vi "Curtin1_AddSettings.vi"(8 "Date?":bool, 9 "Check?":enum16{"Ignore", "Check", "Replace"}(ring)=enum."Check", 10 "Template":string, 11 "Settings in":T2={"Name of test"="", "Date"=timestamp(0 s since 1904-01-01), "Location"="", "Template"="", "Soundcard"="", "resolution"=0, "Sampling rate"=0, "Ch1 Gain "=25.0, "Ch2 Gain"=10.0, "Sample time (s)"=0.0, "Pre-trigger (s)"=0.0, "Hammer Threshold"=0.0, "Positions"=0, "Taps/Position"=0, "Set Names"="", "Freq resolution"=0.0, "Hammer cutoff"=0.0, "Mic cutoff"=0.0, "Double bounce "=0.0, "Hammer Cal"=0.0, "dB Offset"=0.0, "Accel Cal"=0.0, "Vibrometer Cal"=0.0, "Mic Cal"=0.0, "Output"=0, "Voltage Cal"=1.0, "Vibrometer Port"="ASRL27::INSTR", "Range"=4, "High Pass"=2, "Bandwidth"=4, "X Range"=[], "Y Range"=[], "dB Spread"=0.0, "Trigger"=0, "Ch_1"=25, "Ch_2"=25, "flip?"=FALSE, "60Hz"=FALSE, "Time offset"=0.0, "Piezo Cal"=1.0, "Default Notes"="", "Tom"=FALSE} {"Ch_2" min=1 step=1; "Ch_1" min=1 max=100 step=1; "Trigger" items=["Hammer (force)", "Self-tap", "Spacebar"]; "Bandwidth" items=["1 kHz"=1, "5 kHz"=5, "10 kHz"=10, "25 kHz"=25, "50 kHz"=50, "100 kHz"=100]; "High Pass" items=["Off", "13 Hz", "104 Hz"]; "Range" items=["10 mm/s"=1, "20 mm/s"=2, "50 mm/s"=5, "100 mm/s"=10, "200 mm/s"=20, "500 mm/s"=50, "1 m/s"=100, "2 m/s"=200]; "Output" items=["Accelerometer", "Speed (from acceleration)", "Microphone", "Vibrometer", "Piezo"]; "Voltage Cal" format="%#_13g"; "Ch2 Gain" format="%#_13g"; "Ch1 Gain" format="%#_13g"; "Double bounce" min=0.0; "Mic cutoff" min=0.0 format="%#_4g"; "Hammer cutoff" min=0.0 format="%#_4g"; "Freq resolution" min=0.0; "Pre-trigger (s)" format="%#_13g"; "Date" format="%<%H:%M\n%d/%m/%y>T"; "resolution" items=["16 bit"=16, "24 bit"=24, "32 bit"=32]; "Sampling rate" items=["22050 samp/s"=22050, "44100 samp/s"=44100, "48000 samp/s"=48000]}) -> (0 "text":string, 3 "Settings Out":T2={"Name of test"="", "Date"=timestamp(0 s since 1904-01-01), "Location"="", "Template"="", "Soundcard"="", "resolution"=0, "Sampling rate"=0, "Ch1 Gain "=25.0, "Ch2 Gain"=10.0, "Sample time (s)"=0.0, "Pre-trigger (s)"=0.0, "Hammer Threshold"=0.0, "Positions"=0, "Taps/Position"=0, "Set Names"="", "Freq resolution"=0.0, "Hammer cutoff"=0.0, "Mic cutoff"=0.0, "Double bounce "=0.0, "Hammer Cal"=0.0, "dB Offset"=0.0, "Accel Cal"=0.0, "Vibrometer Cal"=0.0, "Mic Cal"=0.0, "Output"=0, "Voltage Cal"=1.0, "Vibrometer Port"="ASRL27::INSTR", "Range"=4, "High Pass"=2, "Bandwidth"=4, "X Range"=[], "Y Range"=[], "dB Spread"=0.0, "Trigger"=0, "Ch_1"=25, "Ch_2"=25, "flip?"=FALSE, "60Hz"=FALSE, "Time offset"=0.0, "Piezo Cal"=1.0, "Default Notes"="", "Tom"=FALSE} {"Ch_2" min=1 step=1; "Ch_1" min=1 max=100 step=1; "Trigger" items=["Hammer (force)", "Self-tap", "Spacebar"]; "Bandwidth" items=["1 kHz"=1, "5 kHz"=5, "10 kHz"=10, "25 kHz"=25, "50 kHz"=50, "100 kHz"=100]; "High Pass" items=["Off", "13 Hz", "104 Hz"]; "Range" items=["10 mm/s"=1, "20 mm/s"=2, "50 mm/s"=5, "100 mm/s"=10, "200 mm/s"=20, "500 mm/s"=50, "1 m/s"=100, "2 m/s"=200]; "Output" items=["Accelerometer", "Speed (from acceleration)", "Microphone", "Vibrometer", "Piezo"]; "Voltage Cal" format="%#_13g"; "Ch2 Gain" format="%#_13g"; "Ch1 Gain" format="%#_13g"; "Double bounce" min=0.0; "Mic cutoff" min=0.0 format="%#_4g"; "Hammer cutoff" min=0.0 format="%#_4g"; "Freq resolution" min=0.0; "Pre-trigger (s)" format="%#_13g"; "Date" format="%<%H:%M\n%d/%m/%y>T"; "resolution" items=["16 bit"=16, "24 bit"=24, "32 bit"=32]; "Sampling rate" items=["22050 samp/s"=22050, "44100 samp/s"=44100, "48000 samp/s"=48000]})   [LabVIEW 2022 SP3]
uses:
  PreferencesControl.ctl
panel:
  out "x = y?":T1
  # "Hz"
  # "dB"
  # "dB"
  # "sec"
  # "sec"
  # "mV/Pa"
  # "mV/m/s2"
  # "mV/mm/s"
  # "V/N"
  # "sec"
  # "sec"
  # "mV/N"
  # "a.u."
  # "a.u."
  # "sec"
  # "Hz"
  # "dB"
  # "dB"
  # "sec"
  # "sec"
  # "mV/Pa"
  # "mV/m/s2"
  # "mV/mm/s"
  # "V/N"
  # "sec"
  # "sec"
  # "mV/N"
  # "a.u."
  # "a.u."
  # "sec"
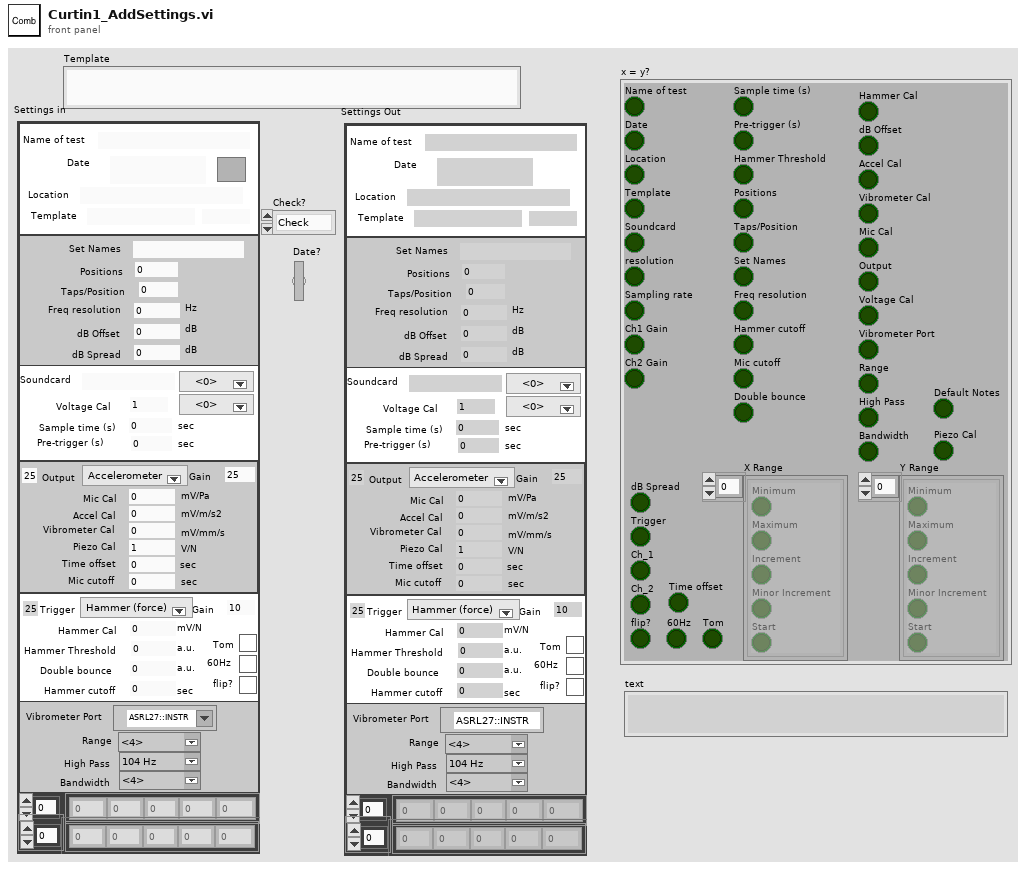
[diagram p1: front panel]
types:
  T1 = cluster{"Name of test":bool, "Date":bool, "Location":bool, "Template":bool, "Soundcard":bool, "resolution":bool, "Sampling rate":bool, "Ch1 Gain ":bool, "Ch2 Gain":bool, "Sample time (s)":bool, "Pre-trigger (s)":bool, "Hammer Threshold":bool, "Positions":bool, "Taps/Position":bool, "Set Names":bool, "Freq resolution":bool, "Hammer cutoff":bool, "Mic cutoff":bool, "Double bounce ":bool, "Hammer Cal":bool, "dB Offset":bool, "Accel Cal":bool, "Vibrometer Cal":bool, "Mic Cal":bool, "Output":bool, "Voltage Cal":bool, "Vibrometer Port":bool, "Range":bool, "High Pass":bool, "Bandwidth":bool, "X Range":cluster{"Minimum":bool, "Maximum":bool, "Increment":bool, "Minor Increment":bool, "Start":bool}[], "Y Range":cluster{"Minimum":bool, "Maximum":bool, "Increment":bool, "Minor Increment":bool, "Start":bool}[], "dB Spread":bool, "Trigger":bool, "Ch_1":bool, "Ch_2":bool, "flip?":bool, "60Hz":bool, "Time offset":bool, "Piezo Cal":bool, "Default Notes":bool, "Tom":bool}
  T2 = typedef "PreferencesControl.ctl" = cluster{"Name of test":string, "Date":timestamp, "Location":string, "Template":string, "Soundcard":string, "resolution":u16, "Sampling rate":u16, "Ch1 Gain ":dbl, "Ch2 Gain":dbl, "Sample time (s)":dbl, "Pre-trigger (s)":dbl, "Hammer Threshold":dbl, "Positions":i16, "Taps/Position":i16, "Set Names":string, "Freq resolution":dbl, "Hammer cutoff":dbl, "Mic cutoff":dbl, "Double bounce ":dbl, "Hammer Cal":dbl, "dB Offset":dbl, "Accel Cal":dbl, "Vibrometer Cal":dbl, "Mic Cal":dbl, "Output":u16, "Voltage Cal":dbl, "Vibrometer Port":refnum<visa-resource-name>, "Range":u16, "High Pass":u16, "Bandwidth":u16, "X Range":cluster{"Minimum":dbl, "Maximum":dbl, "Increment":dbl, "Minor Increment":dbl, "Start":dbl}[], "Y Range":cluster{"Minimum":dbl, "Maximum":dbl, "Increment":dbl, "Minor Increment":dbl, "Start":dbl}[], "dB Spread":dbl, "Trigger":u16, "Ch_1":u8, "Ch_2":u8, "flip?":bool, "60Hz":bool, "Time offset":dbl, "Piezo Cal":dbl, "Default Notes":string, "Tom":bool}
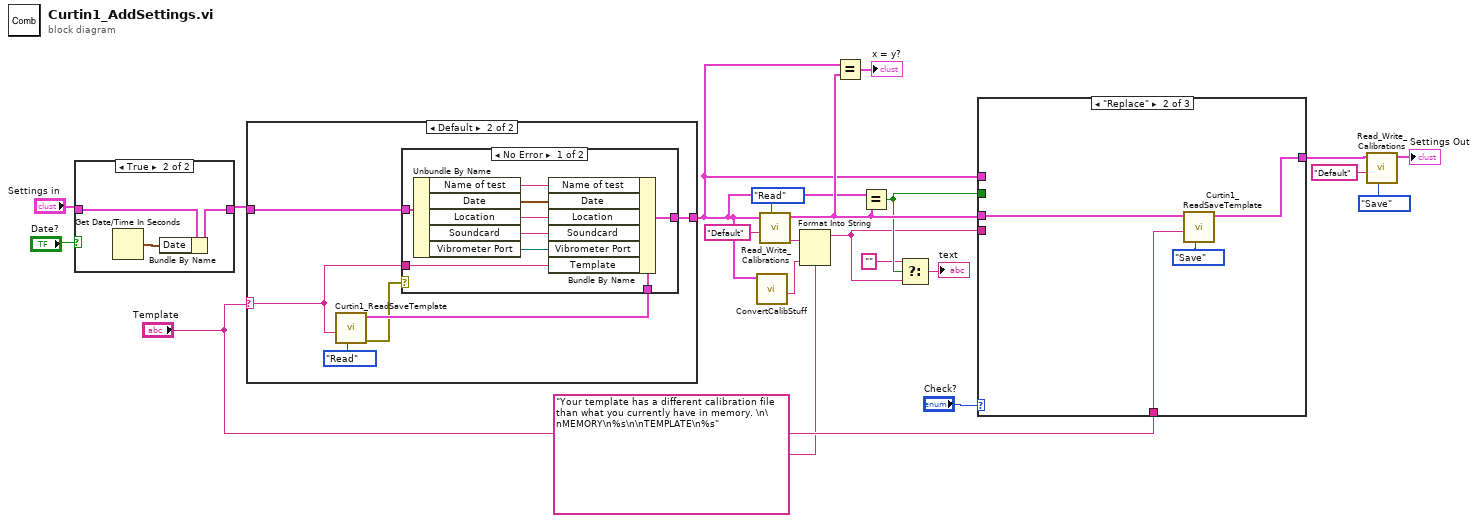
[diagram p0: block diagram]
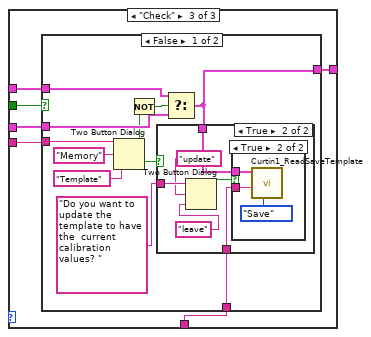
[diagram p3: hidden frame]
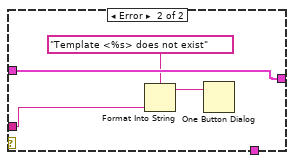
[diagram p9: hidden frame]
diagram:
  n1 = case shown="True" "Date?" {
    tunnel: "Settings in" -> [w22 w24]
    tunnel: [w22 w23] -> w18
    frame False {
    }
    frame True {
      n2 = Get Date/Time In Seconds() -> (seconds since 1Jan1904=w25:timestamp)
      n3 = Bundle By Name(cluster=w24, "Date"=w25) -> (w23:T2)
    }
  }
  n4 = case shown="Default" "Template" {
    selector: "Template" -> [_ w28]
    tunnel: [w26 w32] -> w8
    tunnel: w18 -> [w26 w31]
    frame "" {
    }
    frame Default {
      n5 = call "Curtin1_ReadSaveTemplate.vi"("Task"=enum16{"Save", "Read", "List"}."Read", "Template"=w28) -> ("error out"=w27:errorcluster, "Settings out"=w29:T2)  [unwired: 6 in, 2 out]
      n6 = case shown="No Error" w27 {
        tunnel: [w38 w45] -> w32
        tunnel: w31 -> [w36 w45]
        tunnel: w29 -> [w35 _]
        tunnel: w28 -> [w34 w44]
        frame No Error {
          n7 = Unbundle By Name(w36) -> ("Name of test"=w41:string, "Date"=w40:timestamp, "Location"=w39:string, "Soundcard"=w37:string, "Vibrometer Port"=w33:refnum<visa-resource-name>)
          n8 = Bundle By Name(cluster=w35, "Name of test"=w41, "Date"=w40, "Location"=w39, "Soundcard"=w37, "Vibrometer Port"=w33, "Template"=w34) -> (w38:T2)
        }
        frame Error {
          n9 = Format Into String(format string="Template <%s> does not exist", w44) -> (resulting string=w43:string)  [unwired: 2 in, 1 out]
          n10 = One Button Dialog(message=w43) -> ()  [unwired: 1 in, 1 out]
        }
      }
    }
  }
  n11 = call "ConvertCalibStuff.vi"("Settings in"=w8) -> ("Text"=w5:string)  [unwired: 7 in, 3 out]
  n12 = call "Read_Write_Calibrations.vi"("Task"=enum16{"Save", "Read", "List"}."Read", "Calibration name"="Default", "Settings in"=w8) -> ("file"=w6:string, "Settings out"=w16:T2)  [unwired: 6 in, 1 out]
  n13 = Format Into String(format string="Your template has a different calibration file than what you currently have in memory. \n\nMEMORY\n%s\n\nTEMPLATE\n%s", w6, w5) -> (resulting string=w3:string)  [unwired: 2 in, 1 out]
  n14 = Equal?(x=w8, y=w16) -> (x = y?=→"x = y?":T1)
  n15 = Equal?(x=w8, y=w16) -> (x = y?=w4:bool)
  n16 = Select(t="", s=w4, f=w3) -> (s? t:f=→"text":string)
  n17 = case shown="\"Replace\"" "Check?" {
    tunnel: [w46 w48 w56] -> w10
    tunnel: "Template" -> [_ w47 w55]
    tunnel: w8 -> [w46 _ w54]
    tunnel: w16 -> [_ w49 w53]
    tunnel: w3 -> [_ _ w52]
    tunnel: w4 -> [_ _ w51]
    frame "Ignore", Default {
    }
    frame "Replace" {
      n18 = call "Curtin1_ReadSaveTemplate.vi"("Task"=enum16{"Save", "Read", "List"}."Save", "Template"=w47, "Settings"=w49) -> ("Settings out"=w48:T2)  [unwired: 5 in, 3 out]
    }
    frame "Check" {
      n19 = case shown="False" w51 {
        tunnel: [w58 w76] -> w56
        tunnel: w53 -> [w66 _]
        tunnel: w54 -> [w65 w76]
        tunnel: w52 -> [w63 _]
        tunnel: w55 -> [w57 _]
        frame False {
          n20 = Two Button Dialog(message=w63, 1:"Template" ("F button name (\"Cancel\")"), 2:"Memory" ("T button name (\"OK\")")) -> (T button?=w60:bool)
          n21 = Not(x=w60) -> (.not. x?=w64:bool)
          n22 = Select(t=w65, s=w64, f=w66) -> (s? t:f=w58:T2)
          n23 = case shown="True" w60 {
            tunnel: "Do you want to update the template to have the  current calibration values? " ("T button name (\"OK\")") -> [_ w72]
            tunnel: w58 -> [_ w70]
            tunnel: w57 -> [_ w69]
            frame False {
            }
            frame True {
              n24 = Two Button Dialog(message=w72, 1:"leave" ("F button name (\"Cancel\")"), 2:"update" ("F button name (\"Cancel\")")) -> (T button?=w71:bool)
              n25 = case shown="True" w71 {
                tunnel: w70 -> [_ w74]
                tunnel: w69 -> [_ w73]
                frame False {
                }
                frame True {
                  n26 = call "Curtin1_ReadSaveTemplate.vi"("Task"=enum16{"Save", "Read", "List"}."Save", "Template"=w73, "Settings"=w74) -> ()  [unwired: 5 in, 4 out]
                }
              }
            }
          }
        }
        frame True {
        }
      }
    }
  }
  n27 = call "Read_Write_Calibrations.vi"("Task"=enum16{"Save", "Read", "List"}."Save", "Calibration name"="Default", "Settings in"=w10) -> ("Settings out"=→"Settings Out":T2)  [unwired: 6 in, 2 out]
